vi "C4Buf_release.vi"(0 "c4buf in":refnum<k24>, 11 "error in (no error)":errorcluster) -> (15 "error out":errorcluster)   [LabVIEW 2015, in "libC4HdlLV.lvlib"]
uses:
  libC4HdlLV.lvlib
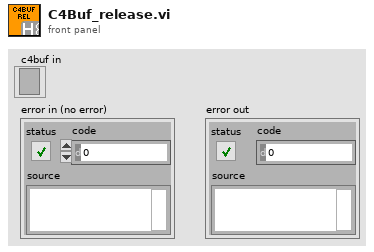
[diagram p1: front panel]
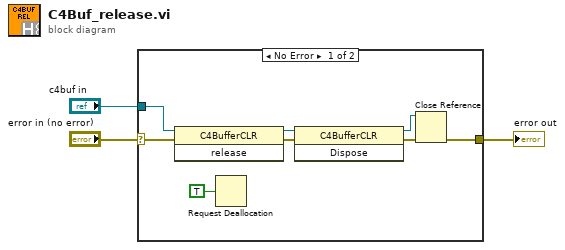
[diagram p0: block diagram]
diagram:
  n1 = case shown="No Error" "error in (no error)" {
    selector: "error in (no error)" -> [w4 w12]
    tunnel: "c4buf in" -> [w10 _]
    tunnel: [w5 w12] -> w3
    frame No Error {
      n2 = invoke class="C4BufferCLR" method="release"(reference=w10, error in=w4) -> (reference out=w9:refnum<k24>, error out=w7:errorcluster)  [unwired: 1 in, 1 out]
      n3 = Request Deallocation(TRUE ("flag")) -> ()
      n4 = invoke class="C4BufferCLR" method="Dispose"(reference=w9, error in=w7) -> (reference out=w8:refnum<k24>, error out=w6:errorcluster)  [unwired: 1 in, 1 out]
      n5 = Close Reference(reference=w8, error in (no error)=w6) -> (error out=w5:errorcluster)
    }
    frame Error {
    }
  }
  "error out" <- w3
